vi "ConvertClusterToByteArr.vi"(7 "data type":enum16{"string", "unsign int"}(ring), 11 "element":variant caption="원소") -> (3 "byte arr":u8[](array[numeric]))   [LabVIEW 2018, in "Library-DataConvert.lvlib"]
uses:
  Library-DataConvert.lvlib
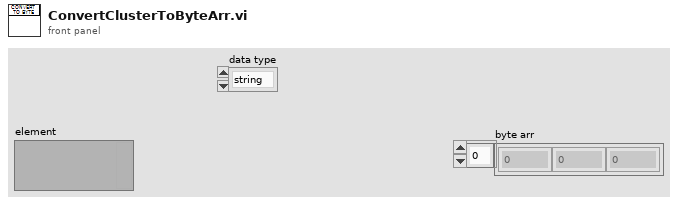
[diagram p1: front panel]
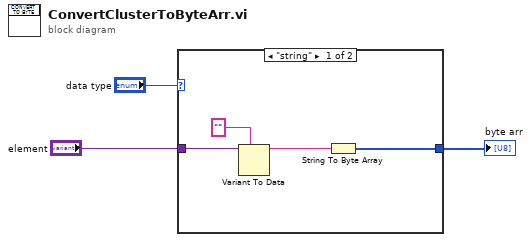
[diagram p0: block diagram]
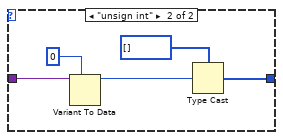
[diagram p2: hidden frame]
diagram:
  n1 = case shown="\"string\"" "data type" {
    tunnel: "element" -> [w7 w12]
    tunnel: [w4 w9] -> w1
    frame "string" {
      n2 = Variant To Data(type="", Variant=w7) -> (data=w5:string)  [unwired: 1 in, 1 out]
      n3 = String To Byte Array(string=w5) -> (unsigned byte array=w4:u8[])
    }
    frame "unsign int" {
      n4 = Variant To Data(type=u32 0, Variant=w12) -> (data=w11:u32)  [unwired: 1 in, 1 out]
      n5 = Type Cast(type=u8[] [], x=w11) -> (*(type *) &x=w9:u8[])
    }
  }
  "byte arr" <- w1
